vi "To Double.vi"(8 "error in (no error)":errorcluster, 11 "Double Scalar SensorData in":refnum<class "Double Scalar SensorData.lvclass">) -> (0 "error out":errorcluster, 2 "Value":dbl, 3 "Double Scalar SensorData out":refnum<class "Double Scalar SensorData.lvclass">)   [LabVIEW 2012, in "Sensor Definition.lvlib" / "Double Scalar SensorData.lvclass"]
uses:
  Double Scalar SensorData.lvclass
  Double Scalar SensorData.lvclass/Double Scalar SensorData.ctl
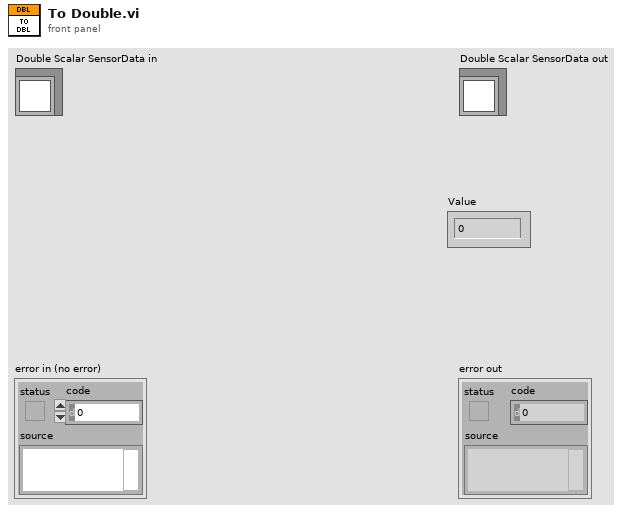
[diagram p1: front panel]
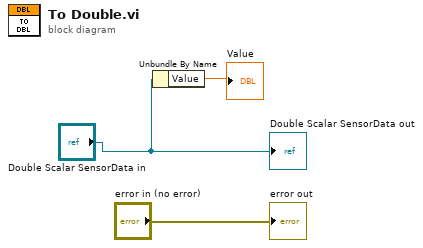
[diagram p0: block diagram]
diagram:
  n1 = Unbundle By Name("Double Scalar SensorData in") -> ("Value"=→"Value":dbl)
  "error out" <- "error in (no error)"
  "Double Scalar SensorData out" <- "Double Scalar SensorData in"
